vi "Enqueue (Single).vi"(4 "timeout in ms (-1)":i32=-1, 6 "Priority Message? Array":bool, 8 "error in (no error)":errorcluster, 9 "Message Data Array":variant, 10 "States":T2=enum."Initialize", 11 "Message Queue":T1) -> (0 "error out":errorcluster, 3 "dup Message Queue":T1)   [LabVIEW 2019, in "Message Queue.lvlib"]
doc: "For a regular message, enqueue the message. For a priority message, enqueue it at the front of the queue."
uses:
  Message Queue.lvlib
  State Name.ctl
  Shared/TypeDefs/Message Queue Ref.ctl
  Shared/TypeDefs/Message Queue Type.ctl
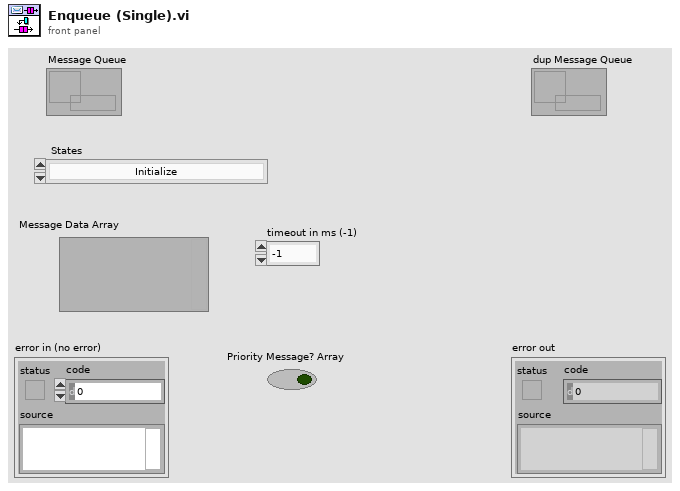
[diagram p1: front panel]
types:
  T1 = typedef "Message Queue Ref.ctl" = refnum<queue>
  T2 = typedef "Message Queue.lvlib/State Name.ctl" = enum16{"Default", "Initialize", "Initialize Data", "Initialize Modules", "Initialize Panel", "Close FP", "Open FP", "Initialize Menu", "Mode", "Update Subpanel", "Error", "Open Help", "About", "Open WebResources", "Exit"}
  T3 = typedef "Message Queue Type.ctl" = cluster{"Custom State Name":string, "Defined State Name":variant, "Call Chain":string[], "Message Data":variant}
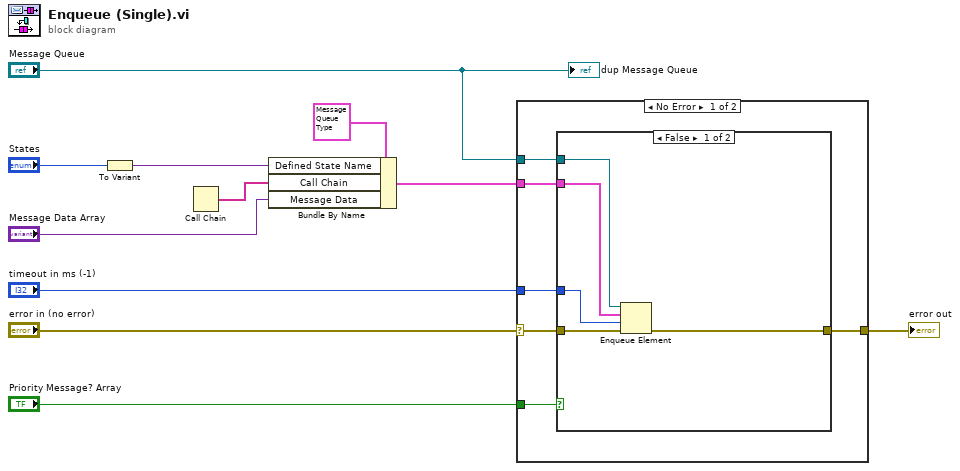
[diagram p0: block diagram]
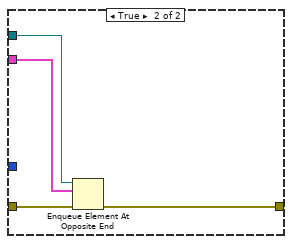
[diagram p2: hidden frame]
diagram:
  n1 = To Variant(anything="States") -> (Variant=w2:variant)
  n2 = Call Chain() -> (call chain=w6:string[])
  n3 = Bundle By Name(cluster=T3 {"Custom State Name"="", "Defined State Name"=variant(enum16{"Default", "Initialize", "Initialize Data", "Initialize Modules", "Initialize Panel", "Close FP", "Open FP", "Initialize Menu", "Mode", "Update Subpanel", "Error", "Open Help", "About", "Open WebResources", "Exit"} enum."Initialize"), "Call Chain"=[], "Message Data"=variant} ("Message Cluster"), "Defined State Name"=w2, "Call Chain"=w6, "Message Data"="Message Data Array") -> (w7:T3)
  n4 = case shown="No Error" "error in (no error)" {
    selector: "error in (no error)" -> [w12 w27]
    tunnel: "Priority Message? Array" -> [w17 _]
    tunnel: [w16 w27] -> w10
    tunnel: "Message Queue" -> [w15 _]
    tunnel: "timeout in ms (-1)" -> [w14 _]
    tunnel: w7 -> [w13 _]
    frame No Error {
      n5 = case shown="False" w17 {
        tunnel: w12 -> [w22 w26]
        tunnel: [w21 w25] -> w16
        tunnel: w15 -> [w20 w24]
        tunnel: w13 -> [w19 w23]
        tunnel: w14 -> [w18 _]
        frame False {
          n6 = Enqueue Element(queue=w20, element=w19, timeout in ms (-1)=w18, error in (no error)=w22) -> (error out=w21:errorcluster)  [unwired: 2 out]
        }
        frame True {
          n7 = Enqueue Element At Opposite End(queue=w24, element=w23, error in (no error)=w26) -> (error out=w25:errorcluster)  [unwired: 1 in, 2 out]
        }
      }
    }
    frame Error {
    }
  }
  "error out" <- w10
  "dup Message Queue" <- "Message Queue"
